vi "External_Highlight Execution.vi"(8 "error in":errorcluster, 9 "Highlight Execution?":bool, 10 "VIs":string[](array[string]), 11 "Application in":refnum<vi>) -> (0 "error out":errorcluster)   [LabVIEW 2013]
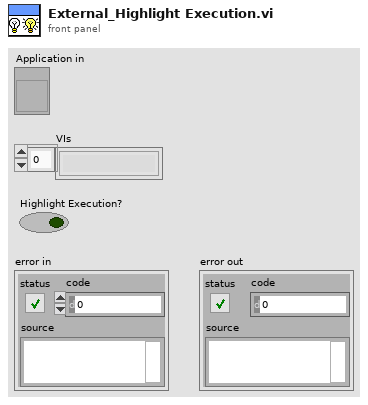
[diagram p1: front panel]
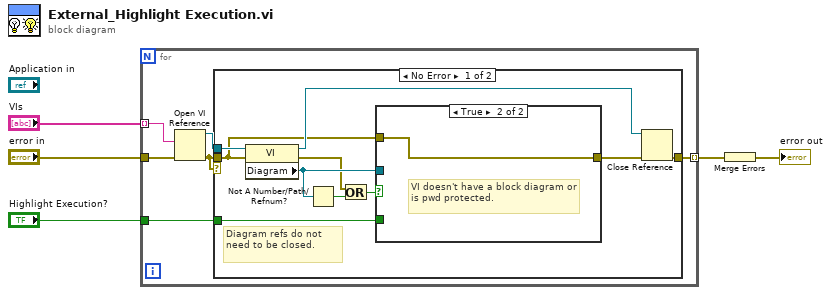
[diagram p0: block diagram]
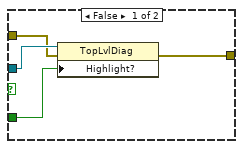
[diagram p2: hidden frame]
diagram:
  n1 = for {
    tunnel: "VIs" -> [w9] mode=indexing
    tunnel: "Highlight Execution?" -> [w7]
    tunnel: "error in" -> [w10]
    tunnel: [w11] -> w3 mode=indexing
    n2 = Open VI Reference(vi path=w9, error in (no error)=w10) -> (vi reference=w8:refnum<vi>, error out=w6:errorcluster)  [unwired: 4 out]
    n3 = case shown="No Error" w6 {
      tunnel: [w21 _] -> w11
      tunnel: w8 -> [w20 _]
      tunnel: w7 -> [w18 _]
      tunnel: w6 -> [w12 _]
      frame No Error {
        # "Diagram refs do not need to be closed."
        n4 = property class="VI"(reference=w20, error in=w12) -> (reference out=w15:refnum<vi>, error out=w13:errorcluster, "Diagram"=w17:refnum<vi>)
        n5 = Not A Number/Path/Refnum?(number/path/refnum=w17) -> (NaN/Path/Refnum?=w16:bool)
        n6 = Or(x=w13, y=w16) -> (x .or. y?=w14:bool)
        n7 = case shown="True" w14 {
          tunnel: [w25 w26] -> w19
          tunnel: w18 -> [w24 _]
          tunnel: w17 -> [w23 _]
          tunnel: w12 -> [w22 w26]
          frame False {
            n8 = property class="TopLvlDiag"(reference=w23, error in=w22, "Highlight?"=w24) -> (error out=w25:errorcluster)  [unwired: 1 out]
          }
          frame True {
            # "VI doesn't have a block diagram or is pwd protected."
          }
        }
        n9 = Close Reference(reference=w15, error in (no error)=w19) -> (error out=w21:errorcluster)
      }
      frame Error {
        # "This VI is no longer in the memory"
      }
    }
  }
  n10 = Merge Errors(w3) -> (→"error out":errorcluster)
